vi "test1-AllWOrkerNodesShareTheSameData.vi"(8 "error in (no error)":errorcluster, 11 "TestCase in":refnum<class "testcase-CSMWorkerMode.lvclass">) -> (0 "error out":errorcluster, 3 "TestCase out":refnum<class "testcase-CSMWorkerMode.lvclass">)   [LabVIEW 2017, in "testcase-CSMWorkerMode.lvclass"]
uses:
  testcase-CSMWorkerMode.lvclass
  src/user.lib/_NEVSTOP/Communicable State Machine(CSM)/_Support/Typedef/_CSM_MODE.ctl
  9c2ff45f-acc9-407c-894c-164613e63933.vi
  <vilib>/addons/_JKI Toolkits/VI Tester/TestCase.llb/TestCase.lvclass
  src/user.lib/_NEVSTOP/Communicable State Machine(CSM)/Communicable State Machine.lvlib
  CSM/CSM-Testcase.lvlib
  C:/Program Files (x86)/National Instruments/LabVIEW 2017/vi.lib/addons/_JKI Toolkits/VI Tester/TestCase.llb/TestCase.lvclass
panel:
  out "LoopCount":i32
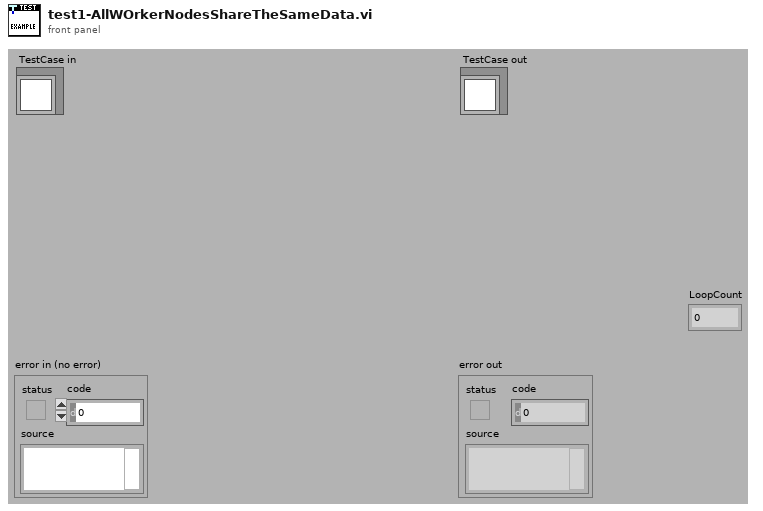
[diagram p1: front panel]
types:
  T1 = typedef "Communicable State Machine.lvlib/_CSM_MODE.ctl" = enum16{"Not Exist", "Stand Alone", "CSM", "Worker", "Worker Agent", "Chain Node", "Chain"}
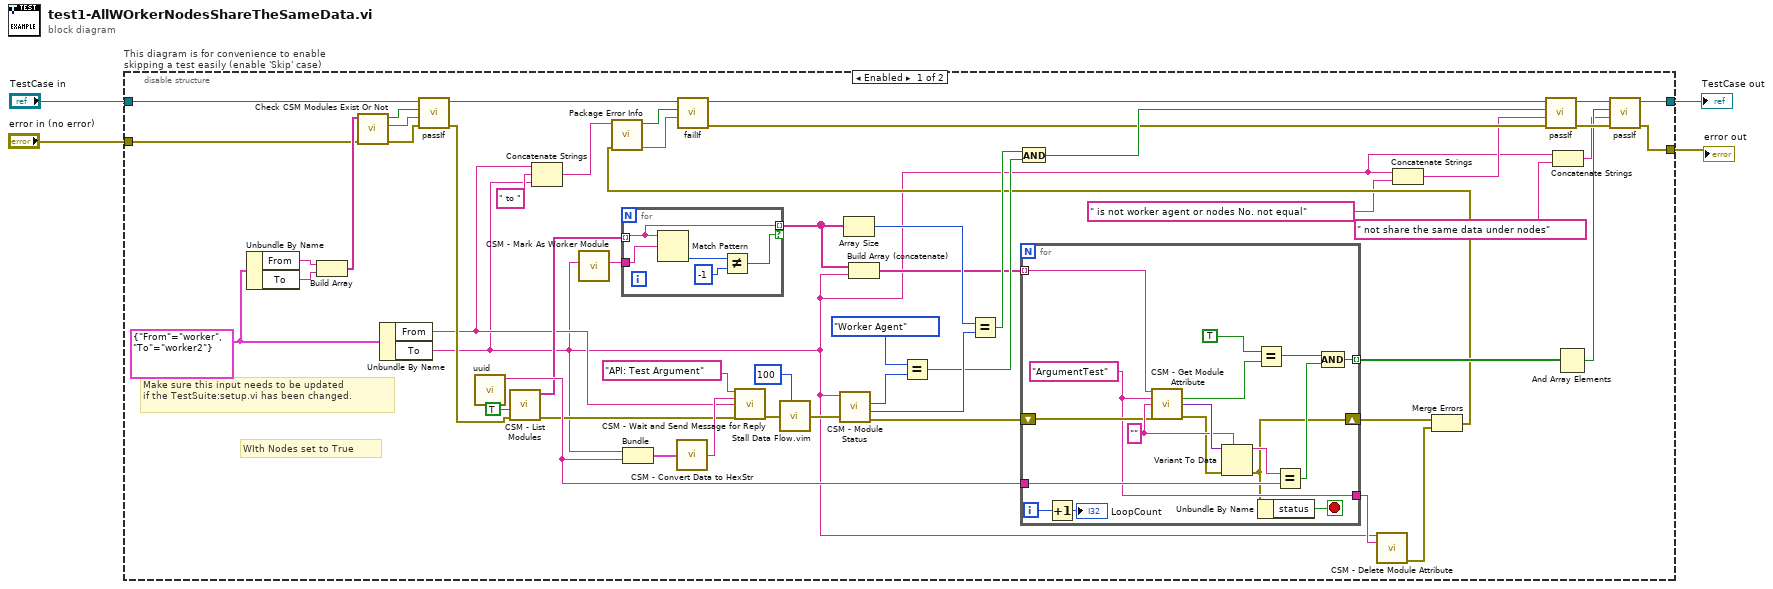
[diagram p0: block diagram]
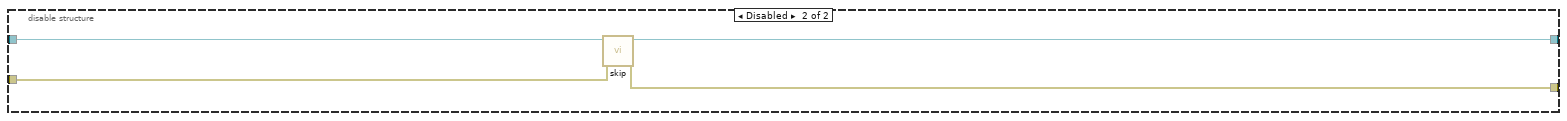
[diagram p2: hidden frame]
diagram:
  n1 = disable-structure "This diagram is for convenience to enable skipping a test easily (enable 'Skip' case)" shown="Enabled" {
    disable-tunnel: "TestCase in" -> [w18 w84]
    disable-tunnel: [w39 w82] -> w1
    disable-tunnel: [w37 w83] -> w3
    disable-tunnel: "error in (no error)" -> [w19 w81]
    frame Enabled {
      w26 = cluster{"From":string, "To":string} {"From"="worker", "To"="worker2"} ("Cluster")
      # "Make sure this input needs to be updated \nif the TestSuite:setup.vi has been changed."
      # "WIth Nodes set to True"
      n2 = Unbundle By Name(w26) -> ("From"=w21:string, "To"=w22:string)
      n3 = Build Array(w21, w22) -> (w20:string[])
      n4 = call "Check CSM Modules Exist Or Not.vi"("error in"=w19, "CSM names in"=w20) -> ("error out"=w23:errorcluster, "Debug string"=w24:string, "All Modules Exist?"=w25:bool)  [unwired: 7 in]
      n5 = Unbundle By Name(w26) -> ("From"=w15:string, "To"=w7:string)
      n6 = call-dynamic "passIf.vi"("error in (no error)"=w23, "message (\"\")"=w24, "pass"=w25, "TestCase in"=w18) -> ("error out"=w17:errorcluster, "TestCase out"=w12:refnum<class "testcase-CSMWorkerMode.lvclass">)  [unwired: 6 in]
      n7 = call "uuid.vi"() -> ("UUID"=w53:string)  [unwired: 11 in]
      n8 = call "CSM - List Modules.vi"("Error In"=w17, "With Nodes? (F)"=TRUE) -> ("error out"=w47:errorcluster, "Module Names"=w50:string[])  [unwired: 8 in]
      n9 = Concatenate Strings(w15, " to " ("string"), w7) -> (w13:string)
      n10 = call "CSM - Mark As Worker Module.vi"("CSM Name"=w7) -> ("CSM Name (Marked As Worker)"=w46:string)  [unwired: 9 in]
      n11 = for {
        tunnel: w50 -> [w78] mode=indexing
        tunnel: [w78] -> w36 mode=indexing if=w77
        tunnel: w46 -> [w76]
        n12 = Match Pattern(string=w78, regular expression=w76) -> (offset past match=w80:i32)  [unwired: 1 in, 3 out]
        n13 = Not Equal?(x=w80, y=-1) -> (x != y?=w77:bool)
      }
      n14 = Bundle("To"=w7, "UUID"=w53) -> (w55:cluster{"To":string, "UUID":string})  [unwired: 1 in]
      n15 = call "CSM - Convert Data to HexStr.vi"("Variant"=w55) -> ("HEX String (0-9,A-F)"=w54:string)  [unwired: 8 in]
      n16 = call "CSM - Wait and Send Message for Reply.vi"("State"="API: Test Argument", "Arguments (\"\")"=w54, "Target Module"=w15, "Error In (No Error)"=w47) -> ("error out"=w57:errorcluster)  [unwired: 8 in, 3 out]
      n17 = call "Stall Data Flow.vim"("value in"=w57, "milliseconds to wait"=u32 100) -> ("value out"=w52:errorcluster)  [unwired: 1 out]
      n18 = call "CSM - Module Status.vi"("Error In"=w52, "CSM Name"=w7) -> ("error out"=w34:errorcluster, "#Nodes"=w45:i32, "Mode"=w48:T1)  [unwired: 5 in, 2 out]
      n19 = Array Size(array=w36) -> (size(s)=w44:i32)
      n20 = Build Array (concatenate)(w36, w7) -> (w35:string[])
      n21 = Equal?(x=_CSM_MODE."Worker Agent" ("Mode 2"), y=w48) -> (x = y?=w42:bool)
      n22 = Equal?(x=w44, y=w45) -> (x = y?=w43:bool)
      n23 = And(x=w43, y=w42) -> (x .and. y?=w41:bool)
      n24 = for {
        tunnel: w53 -> [w75]
        tunnel: w35 -> [w66] mode=indexing
        shift-right: [w60] -> w30
        shift-left: w34 -> [w65]
        tunnel: [w64] -> w33 mode=indexing
        tunnel: [w63] -> w31
        i -> [w62]
        stop <- w59 stop-if-true
        w71 = ""
        w63 = "ArgumentTest" ("Attribute")
        n25 = Increment(x=w62) -> (x+1=→"LoopCount":i32)
        n26 = call "CSM - Get Module Attribute.vi"("CSM Name"=w66, "Attribute"=w63, "Default Value (Empty Variant)"=w71, "Error In"=w65) -> ("Found"=w74:bool, "Value"=w72:variant, "error out"=w69:errorcluster)  [unwired: 7 in, 2 out]
        n27 = Variant To Data(error in=w69, type=w71, Variant=w72) -> (data=w70:string, error out=w60:errorcluster)
        n28 = Equal?(x=TRUE, y=w74) -> (x = y?=w68:bool)
        n29 = Unbundle By Name(w60) -> ("status"=w59:bool)
        n30 = Equal?(x=w70, y=w75) -> (x = y?=w67:bool)
        n31 = Compound Arithmetic op=AND(w68, w67) -> (w64:bool)
      }
      n32 = call "CSM - Delete Module Attribute.vi"("CSM Name"=w7, "Attribute"=w31) -> ("error out"=w29:errorcluster)  [unwired: 10 in, 3 out]
      n33 = Concatenate Strings(w7, " is not worker agent or nodes No. not equal" ("string")) -> (w9:string)
      n34 = Merge Errors(w30, w29) -> (w16:errorcluster)
      n35 = call "Package Error Info.vi"("error in"=w16, "String in"=w13) -> ("packed error info out"=w27:string, "error status"=w28:bool)  [unwired: 8 in]
      n36 = call-dynamic "failIf.vi"("message (\"\")"=w27, "fail"=w28, "TestCase in"=w12) -> ("error out"=w11:errorcluster, "TestCase out"=w10:refnum<class "testcase-CSMWorkerMode.lvclass">)  [unwired: 7 in]
      n37 = call-dynamic "passIf.vi"("error in (no error)"=w11, "message (\"\")"=w9, "pass"=w41, "TestCase in"=w10) -> ("error out"=w38:errorcluster, "TestCase out"=w40:refnum<class "testcase-CSMWorkerMode.lvclass">)  [unwired: 6 in]
      n38 = Concatenate Strings(w7, " not share the same data under nodes" ("string")) -> (w5:string)
      n39 = And Array Elements(Boolean array=w33) -> (logical AND=w32:bool)
      n40 = call-dynamic "passIf.vi"("error in (no error)"=w38, "message (\"\")"=w5, "pass"=w32, "TestCase in"=w40) -> ("error out"=w37:errorcluster, "TestCase out"=w39:refnum<class "testcase-CSMWorkerMode.lvclass">)  [unwired: 6 in]
    }
    frame Disabled {
      # "skip test result while test is under development"
      n41 = call <vilib>:"skip.vi"("error in (no error)"=w81, "TestCase in"=w84) -> ("error out"=w83:errorcluster, "TestCase out"=w82:refnum<class "testcase-CSMWorkerMode.lvclass">)  [unwired: 8 in]
    }
  }
  "error out" <- w3
  "TestCase out" <- w1
